vi "Get Jenkins Configuration.vi"(8 "error in (no error)":errorcluster) -> (0 "error out":errorcluster, 3 "Number of Executors":i32)   [LabVIEW 2014]
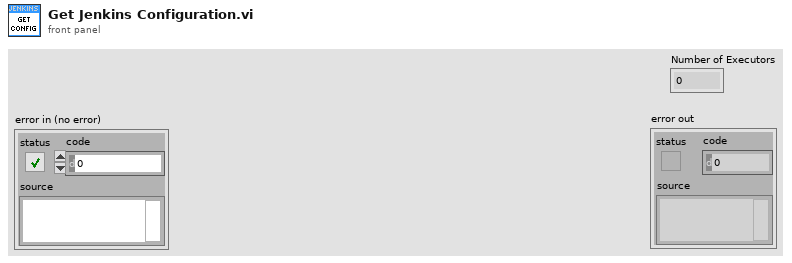
[diagram p1: front panel]
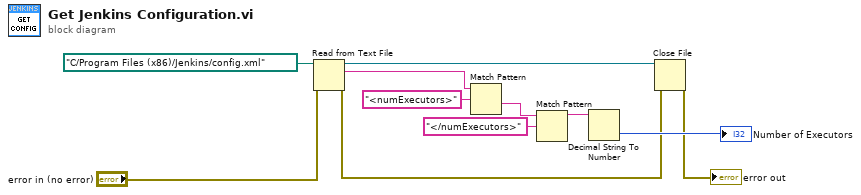
[diagram p0: block diagram]
diagram:
  n1 = Read from Text File(file (use dialog)=path "C:/Program Files (x86)/Jenkins/config.xml" ("XML File Path"), error in="error in (no error)") -> (refnum out=w3:refnum<file>, text=w10:string, error out=w2:errorcluster)  [unwired: 2 in, 1 out]
  n2 = Match Pattern(string=w10, regular expression="<numExecutors>") -> (after substring=w8:string)  [unwired: 1 in, 3 out]
  n3 = Match Pattern(string=w8, regular expression="</numExecutors>") -> (before substring=w5:string)  [unwired: 1 in, 3 out]
  n4 = Decimal String To Number(string=w5) -> (number=→"Number of Executors":i32)  [unwired: 2 in, 1 out]
  n5 = Close File(refnum=w3, error in=w2) -> (error out=→"error out":errorcluster)  [unwired: 1 out]
